vi "Example_SimpleVariableRead.vi"() -> ()   [LabVIEW 2013]
panel:
  out "errorOut":errorcluster
  in  "serialNumber":string="0NODCNPP"
  in  "partNumber":string="SD-PXE-DIO-H0002-1G"
  out "variableValue":i32
  in  "stop":bool
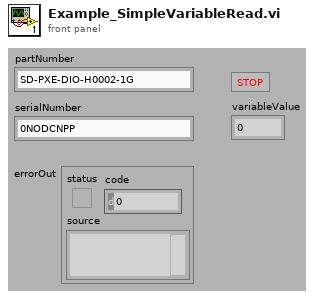
[diagram p1: front panel]
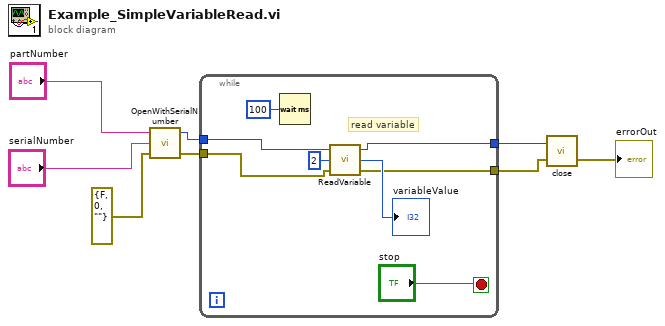
[diagram p0: block diagram]
diagram:
  n1 = call <vilib>:"OpenWithSerialNumber.vi"("errorIn"=errorcluster {"status"=FALSE, "code"=0, "source"=""}, "serialNumber"="serialNumber", "partNumber"="partNumber") -> ("errorOut"=w4:errorcluster, "moduleID"=w6:i32)  [unwired: 1 in]
  n2 = while {
    tunnel: w6 -> [w14]
    tunnel: [w13] -> w1
    tunnel: w4 -> [w10]
    tunnel: [w9] -> w2
    stop <- "stop" stop-if-true
    # "read variable"
    n3 = Wait (ms)(milliseconds to wait=u32 100) -> ()  [unwired: 1 out]
    n4 = call <vilib>:"ReadVariable.vi"("errorIn"=w10, "Number"=2, "ModuleID"=w14) -> ("errorOut"=w9:errorcluster, "variableValue"=→"variableValue":i32, "ModuleIDOut"=w13:i32)
  }
  n5 = call <vilib>:"close.vi"("errorIn"=w2, "moduleID"=w1) -> ("errorOut"=→"errorOut":errorcluster)  [unwired: 1 in]
